vi "LocalStorage.vi"() -> ()   [LabVIEW 2017]
uses:
  <vilib>/Platform/browser.llb/Open URL in Default Browser (string).vi
  <userlib>/Simple XML/_polymorphics/Create Tag - Root.vi
  <userlib>/Simple XML/_polymorphics/Create Tag - Child.vi
  <userlib>/Simple XML/_polymorphics/Create Tag - Child with Text.vi
  <userlib>/Simple XML/Simple XML.lvlib
  <vilib>/xml/NI_XML.lvlib
panel:
  out "ALERT":bool
  in  "stop":bool
  in  "dA":dbl(slide) scale=0.0..300.0
  in  "dB":dbl(slide) scale=0.0..300.0
  in  "dC":dbl(slide) scale=0.0..300.0
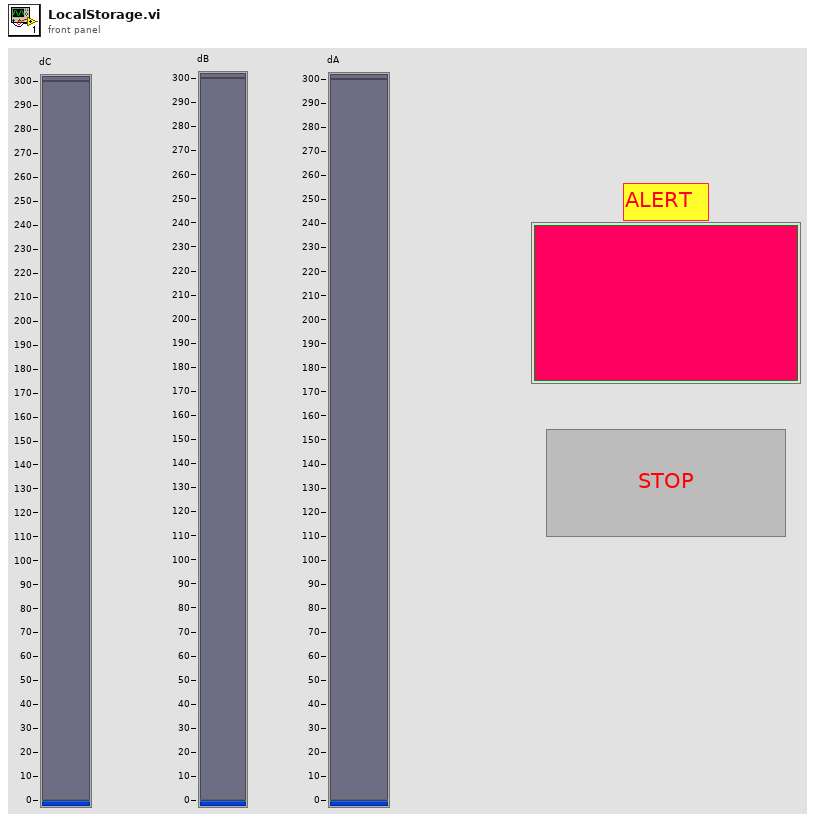
[diagram p1: front panel]
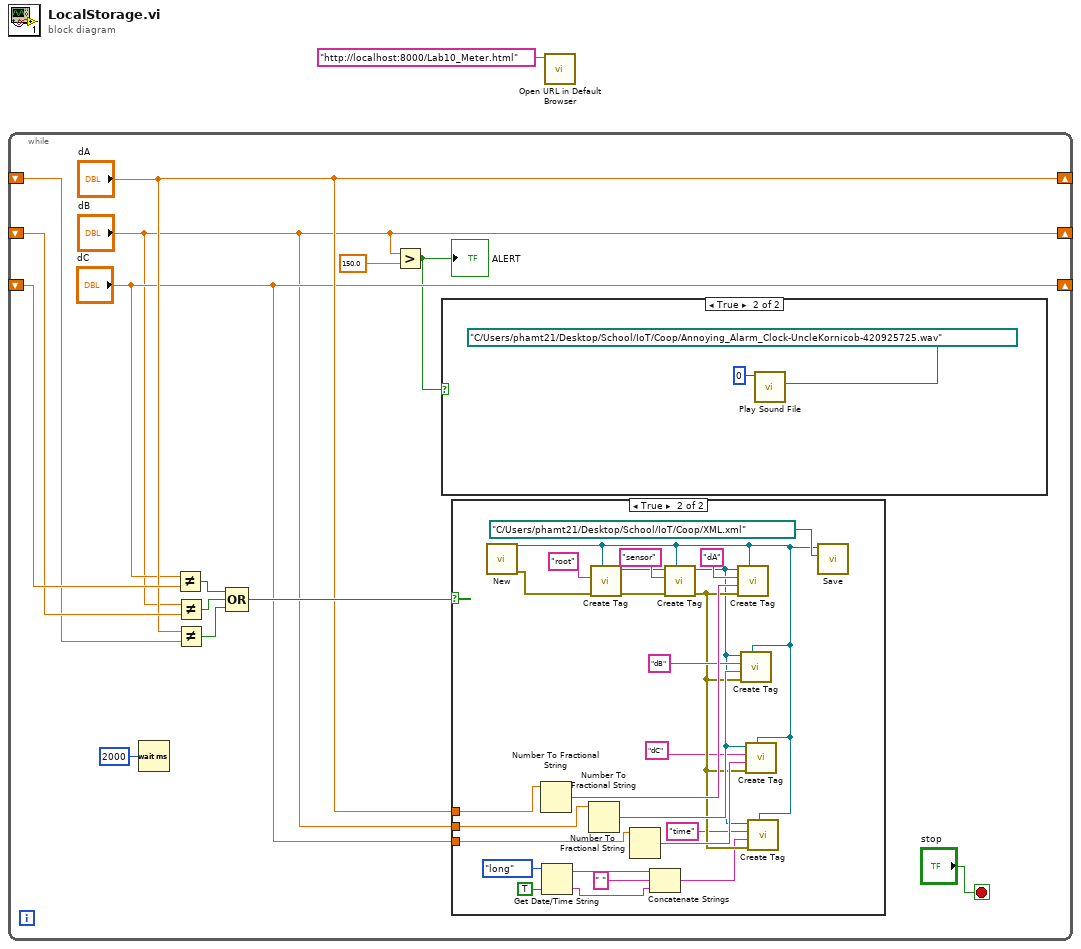
[diagram p0: block diagram]
diagram:
  n1 = while {
    shift-right: ["dC"] -> _
    shift-left: _ -> [w15]
    shift-right: ["dB"] -> _
    shift-left: _ -> [w10]
    shift-right: ["dA"] -> _
    shift-left: _ -> [w9]
    stop <- "stop" stop-if-true
    n2 = Wait (ms)(milliseconds to wait=u32 2000) -> ()  [unwired: 1 out]
    n3 = Not Equal?(x="dC", y=w15) -> (x != y?=w14:bool)
    n4 = Not Equal?(x="dB", y=w10) -> (x != y?=w13:bool)
    n5 = Not Equal?(x="dA", y=w9) -> (x != y?=w12:bool)
    n6 = Compound Arithmetic op=OR(w14, w13, w12) -> (w11:bool)
    n7 = Greater?(x="dB", y=150.0) -> (0:w3:bool)
    "ALERT" <- w3
    n8 = case shown="True" w3 {
      frame False {
      }
      frame True {
        n9 = call <vilib>:"Play Sound File.vi"("path"=path "C:/Users/phamt21/Desktop/School/IoT/Coop/Annoying_Alarm_Clock-UncleKornicob-420925725.wav", "device ID"=u32 0) -> ()  [unwired: 8 in, 2 out]
      }
    }
    n10 = case shown="True" w11 {
      tunnel: "dC" -> [_ w30]
      tunnel: "dB" -> [_ w32]
      tunnel: "dA" -> [_ w36]
      frame False {
      }
      frame True {
        n11 = call <vilib>:"New.vi"() -> ("error out"=w40:errorcluster, "DOM document out"=w18:refnum<k20>)  [unwired: 8 in]
        n12 = Number To Fractional String(number=w36) -> (F-format string=w35:string)  [unwired: 3 in]
        n13 = Get Date/Time String(date format (0)=enum16{"short", "long", "abbreviated"}."long", want seconds? (F)=TRUE) -> (date string=w26:string, time string=w24:string)  [unwired: 1 in]
        n14 = Number To Fractional String(number=w32) -> (F-format string=w31:string)  [unwired: 3 in]
        n15 = call-poly <userlib>:"Create Tag.vi"("DOM document reference"=w18, "error in (no error)"=w40, "Tag Name"="root") -> ("error out"=w39:errorcluster, "Element reference"=w38:refnum<k20>)  [unwired: 7 in]
        n16 = Number To Fractional String(number=w30) -> (F-format string=w29:string)  [unwired: 3 in]
        n17 = Concatenate Strings(w26, " " ("string"), w24) -> (w22:string)
        n18 = call-poly <userlib>:"Create Tag.vi"("DOM Document reference"=w18, "error in (no error)"=w39, "Tag Name"="sensor", "Parent Element reference"=w38) -> ("error out"=w23:errorcluster, "Child Element reference"=w19:refnum<k20>)  [unwired: 6 in]
        n19 = call-poly <userlib>:"Create Tag.vi"("DOM document reference"=w18, "error in (no error)"=w23, "Text Data"=w35, "Tag Name"="dA", "Parent Element reference"=w19) -> ()  [unwired: 5 in, 2 out]
        n20 = call-poly <userlib>:"Create Tag.vi"("DOM document reference"=w18, "error in (no error)"=w23, "Text Data"=w31, "Tag Name"="dB", "Parent Element reference"=w19) -> ()  [unwired: 5 in, 2 out]
        n21 = call-poly <userlib>:"Create Tag.vi"("DOM document reference"=w18, "error in (no error)"=w23, "Text Data"=w29, "Tag Name"="dC", "Parent Element reference"=w19) -> ()  [unwired: 5 in, 2 out]
        n22 = call-poly <userlib>:"Create Tag.vi"("DOM document reference"=w18, "error in (no error)"=w23, "Text Data"=w22, "Tag Name"="time", "Parent Element reference"=w19) -> ()  [unwired: 5 in, 2 out]
        n23 = call <vilib>:"Save.vi"("XML file path"=path "C:/Users/phamt21/Desktop/School/IoT/Coop/XML.xml", "DOM document in"=w18) -> ()  [unwired: 7 in, 3 out]
      }
    }
  }
  n24 = call-poly <vilib>:"Open URL in Default Browser.vi"("URL"="http://localhost:8000/Lab10_Meter.html") -> ()  [unwired: 5 in, 2 out]
